vi "CalcNewVel.vi"(9 "dV Wind":dbl[](array[numeric]), 10 "dV Drag":dbl[](array[numeric]), 11 "Old Robot Velocity":dbl[](array[numeric])) -> (3 "New Robot Velocity":dbl[](array[numeric]))   [LabVIEW 2012]
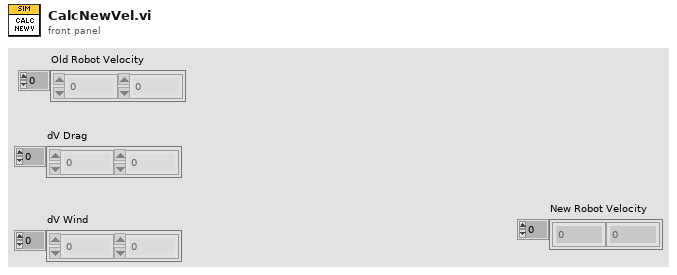
[diagram p1: front panel]
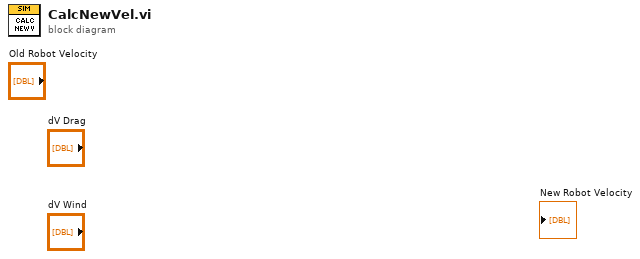
[diagram p0: block diagram]
diagram:
